vi "MAIN.vi"() -> ()   [LabVIEW 2013]
panel:
  out "error out":errorcluster
  out "# of Address Found":i32
  out "Cancelled?":bool
  out "element":string
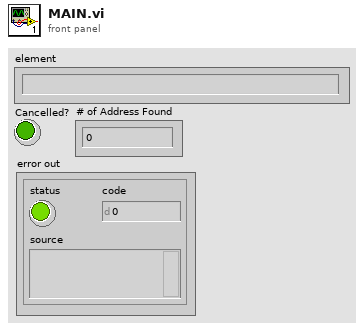
[diagram p1: front panel]
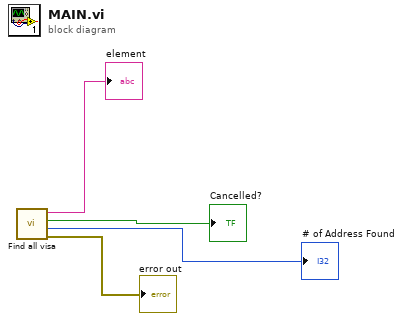
[diagram p0: block diagram]
diagram:
  n1 = call "Find all visa.vi"() -> ("error out"=→"error out":errorcluster, "# of Address Found"=→"# of Address Found":i32, "Cancelled?"=→"Cancelled?":bool, "element"=→"element":string)  [unwired: 8 in]
